vi "ADC.vi"(9 "编码位数L":dbl=8.0, 10 "量化阶Δ(V)":dbl=0.02, 11 "信号数组(V)":dbl[](array[numeric])) -> (3 "编码数组":digitaldata)   [LabVIEW 2018]
uses:
  <vilib>/Waveform/DWDTOps.llb/DWDT Analog to Digital.vi
  <vilib>/Waveform/DWDTOps.llb/DWDT Digital to Binary U32.vi
panel:
  # "输入：信号数组x(t)，量化阶Δ，（二进制）编码位数L（=8）\n输出：编码二进制数组（数字数据）"
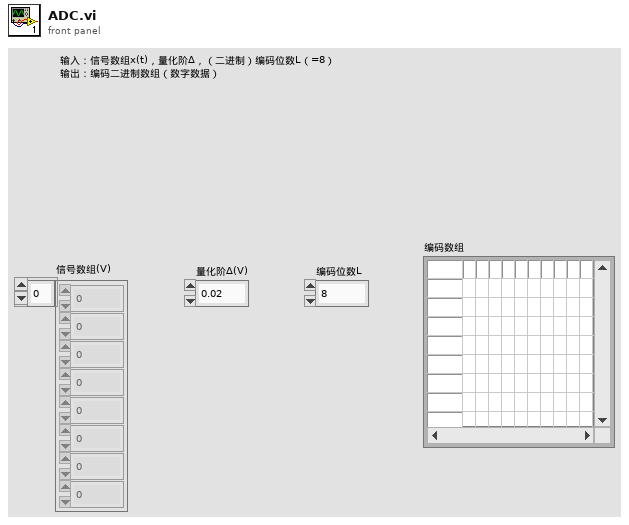
[diagram p1: front panel]
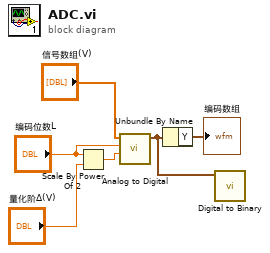
[diagram p0: block diagram]
diagram:
  n1 = Scale By Power Of 2(n="编码位数L", x="量化阶Δ(V)") -> (x*2^n=w5:dbl)
  n2 = call-poly <vilib>:"Analog to Digital.vi"("full-scale range (pk-pk)"=w5, "resolution (16 bit)"="编码位数L", "analog waveform"="信号数组(V)") -> ("digital waveform"=w2:digitalwaveform)  [unwired: 5 in, 3 out]
  n3 = Unbundle By Name ("获取波形成分")(w2) -> ("Y"=→"编码数组":digitaldata)
  n4 = call-poly <vilib>:"Digital to Binary.vi"("digital waveform"=w2) -> ()  [unwired: 9 in, 2 out]
